vi "Read Measurements.vi"(8 "error in":errorcluster, 9 "Data Frame Format In":T1, 10 "Unit ID (A)":string="A", 11 "VISA Session In":refnum<visa-resource-name>="Alicat") -> (0 "error out":errorcluster, 1 "Data Frame Format Out":T1, 2 "Data Cluster":T2, 3 "VISA Session Out":refnum<visa-resource-name>, 4 "Unknown Dataframe Info":bool, 5 "Error/Overrange/Unknown String":string, 6 "Error Present":bool, 7 "Range Exceeded":bool)   [LabVIEW 2020]
doc: "Polls the Alicat device for its data frame and outputs cluster of data, retrieved/used data flags, and error/overrange/unknown indicators and strings. Data is parsed according to data flag inputs, and if none are present the device will query the data flags (adding a considerable amount of time to the VI's execution)."
uses:
  Data Cluster.ctl
  Data Frame.ctl
  <vilib>/Instr/_visa.llb/VISA Flush IO Buffer Mask.ctl
panel:
  # "Totalizer Timer"
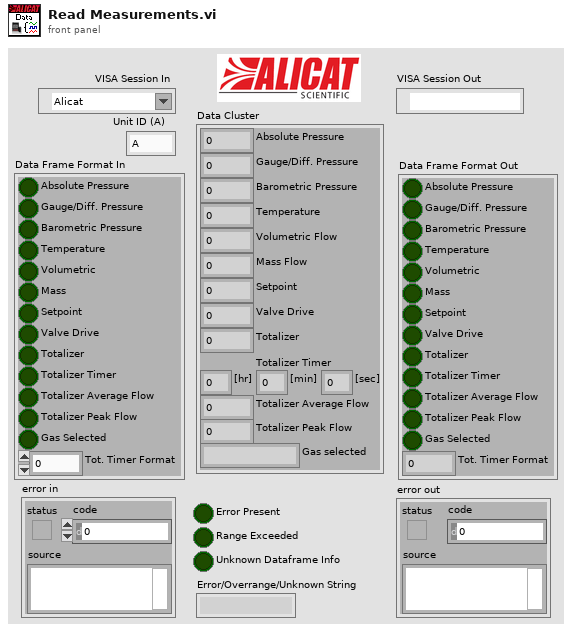
[diagram p1: front panel]
types:
  T1 = typedef "Data Frame.ctl" = cluster{"Absolute Pressure":bool, "Gauge/Diff. Pressure":bool, "Barometric Pressure":bool, "Temperature":bool, "Volumetric":bool, "Mass":bool, "Setpoint":bool, "Valve Drive":bool, "Totalizer":bool, "Totalizer Timer":bool, "Totalizer Average Flow":bool, "Totalizer Peak Flow":bool, "Gas Selected":bool, "Tot. Timer Format":u16}
  T2 = typedef "Data Cluster.ctl" = cluster{"Absolute Pressure":dbl, "Gauge/Diff. Pressure":dbl, "Barometric Pressure":dbl, "Temperature":dbl, "Volumetric Flow":dbl, "Mass Flow":dbl, "Setpoint":dbl, "Valve Drive":dbl, "Totalizer":dbl, "[hr]":dbl, "[min]":dbl, "[sec]":dbl, "Totalizer Average Flow":dbl, "Totalizer Peak Flow":dbl, "Gas selected":string}
  T3 = cluster{"Absolute Pressure":dbl, "Gauge/Diff. Pressure":dbl, "Barometric Pressure":dbl, "Temperature":dbl, "Volumetric":dbl, "Mass":dbl, "Setpoint":dbl, "Valve Drive":dbl, "Totalizer":dbl, "[hr]":dbl, "[min]":dbl, "[sec]":dbl, "Totalizer Average Flow":dbl, "Totalizer Peak Flow":dbl, "Gas selected":string}
  T4 = typedef "VISA Flush IO Buffer Mask.ctl" = u16
  T5 = cluster{"Absolute Pressure":dbl, "Gauge/Diff. Pressure":dbl, "Barometric Pressure":dbl, "Temperature":dbl, "Volumetric Flow":dbl, "Mass Flow":dbl, "Setpoint":dbl, "Valve Drive":dbl, "Totalizer":dbl, "[hr]":dbl, "[min]":dbl, "[sec]":dbl, "Totalizer Average Flow":dbl, "Totalizer Peak Flow":dbl, "Gas selected":string}
  T6 = cluster{"Absolute Pressure":bool, "Gauge/Diff. Pressure":bool, "Barometric Pressure":bool, "Temperature":bool, "Volumetric":bool, "Mass":bool, "Setpoint":bool, "Valve Drive":bool, "Totalizer":bool, "Totalizer Timer":bool, "Totalizer Average Flow":bool, "Totalizer Peak Flow":bool, "Gas Selected":bool, "Tot. Timer Format":u16}
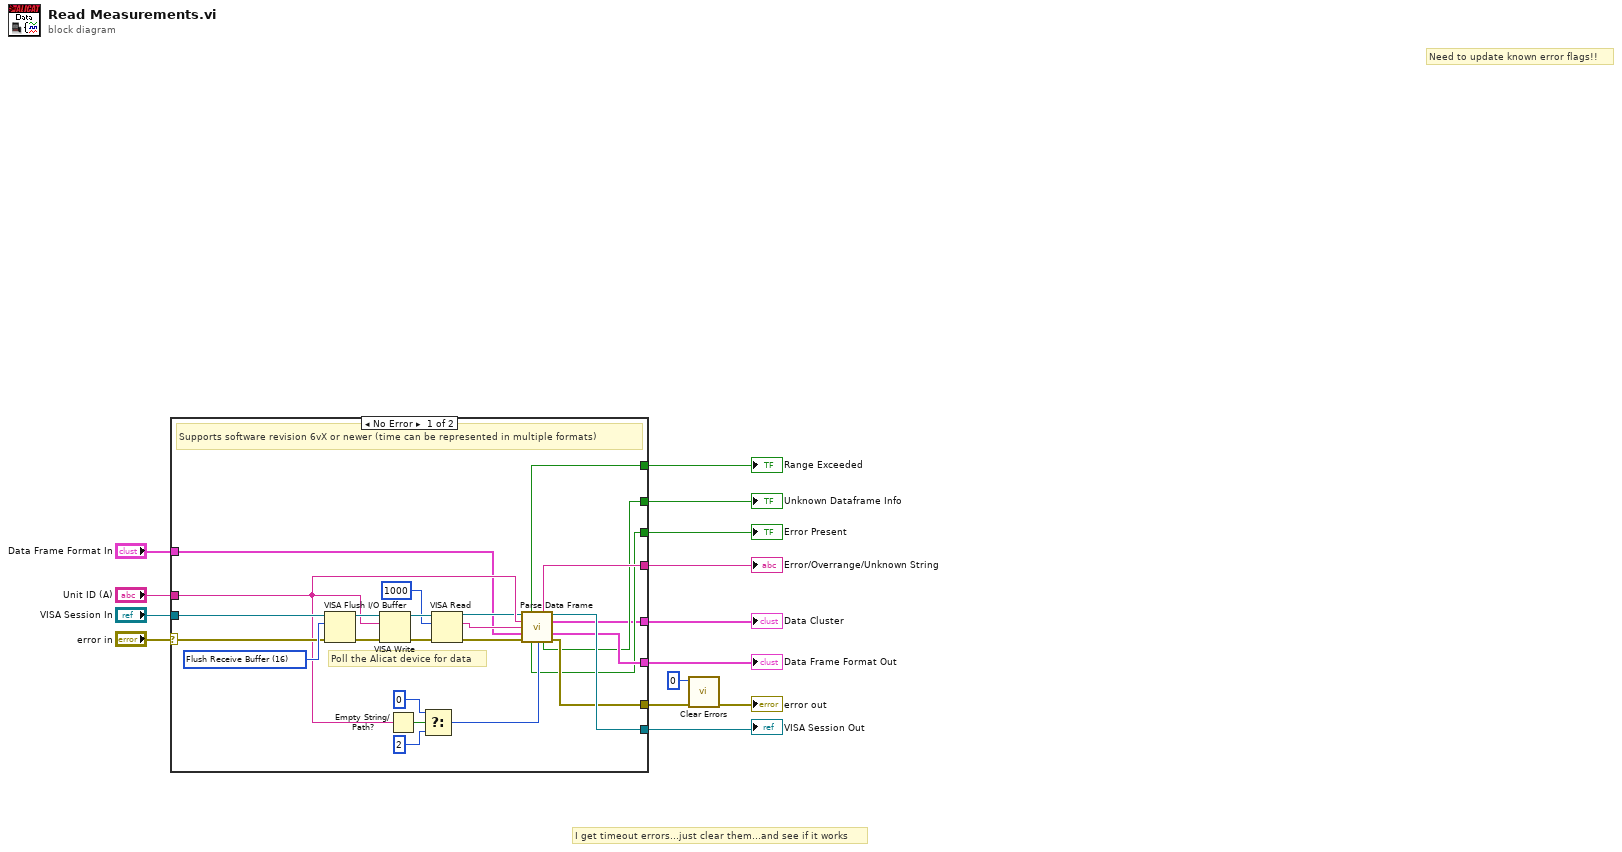
[diagram p0: block diagram]
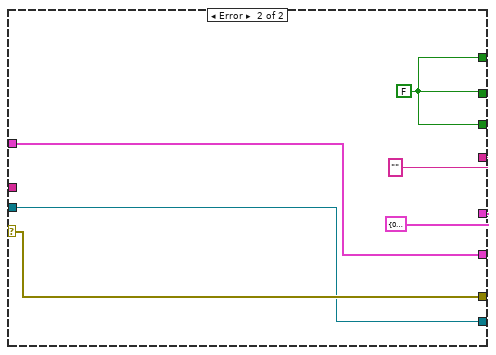
[diagram p2: hidden frame]
diagram:
  # "I get timeout errors...just clear them...and see if it works"
  # "Need to update known error flags!!"
  n1 = case shown="No Error" "error in" {
    selector: "error in" -> [w28 w45]
    tunnel: "VISA Session In" -> [w27 w44]
    tunnel: "Unit ID (A)" -> [w26 _]
    tunnel: [w16 w41] -> w13
    tunnel: [w22 w41] -> w12
    tunnel: [w17 w41] -> w11
    tunnel: [w21 ""] -> w10
    tunnel: [w20 w44] -> w9
    tunnel: [w19 w45] -> w3
    tunnel: "Data Frame Format In" -> [w23 w43]
    tunnel: [w18 w43] -> w5
    tunnel: [w15 T3 {"Absolute Pressure"=0.0, "Gauge/Diff. Pressure"=0.0, "Barometric Pressure"=0.0, "Temperature"=0.0, "Volumetric"=0.0, "Mass"=0.0, "Setpoint"=0.0, "Valve Drive"=0.0, "Totalizer"=0.0, "[hr]"=0.0, "[min]"=0.0, "[sec]"=0.0, "Totalizer Average Flow"=0.0, "Totalizer Peak Flow"=0.0, "Gas selected"=""} ("Data Cluster 2")] -> w8
    frame No Error {
      w34 = T4 16 items=["Flush Receive Buffer"=16, "Write Transmit Buffer to Device"=32, "Flush Receive Buffer (No I/O)"=64, "Flush Transmit Buffer"=128] ("Mask")
      # "Poll the Alicat device for data"
      # "Supports software revision 6vX or newer (time can be represented in multiple formats)"
      n2 = VISA Flush I/O Buffer(VISA resource name=w27, mask (16)=w34, error in (no error)=w28) -> (VISA resource name out=w32:refnum<visa-resource-name>, error out=w30:errorcluster)
      n3 = VISA Write(VISA resource name=w32, write buffer=w26, error in (no error)=w30) -> (VISA resource name out=w33:refnum<visa-resource-name>, error out=w31:errorcluster)  [unwired: 1 out]
      n4 = Empty String/Path?(string/path=w26) -> (empty?=w35:bool)
      n5 = Select(t=u32 0, s=w35, f=u32 2) -> (s? t:f=w38:u32)
      n6 = VISA Read(VISA resource name=w33, byte count=u32 1000, error in (no error)=w31) -> (VISA resource name out=w24:refnum<visa-resource-name>, read buffer=w39:string, error out=w25:errorcluster)  [unwired: 1 out]
      n7 = call "Parse Data Frame.vi"("VISA Session In"=w24, "Unit ID (A)"=w26, "Data Frame Input"=w39, "Data Frame Format In"=w23, "error in"=w25, "Offset (2 if polling, 0 if streaming)"=w38) -> ("Range Exceeded"=w22:bool, "Error/Overrange/Unknown String"=w21:string, "VISA Session Out"=w20:refnum<visa-resource-name>, "Data Cluster"=w15:T5, "Data Frame Format Out"=w18:T6, "Error Present"=w16:bool, "Unknown Dataframe Info"=w17:bool, "error out"=w19:errorcluster)  [unwired: 2 in]
    }
    frame Error {
      w41 = FALSE
    }
  }
  "VISA Session Out" <- w9
  "Error Present" <- w13
  "Range Exceeded" <- w12
  "Unknown Dataframe Info" <- w11
  "Error/Overrange/Unknown String" <- w10
  "Data Cluster" <- w8
  "Data Frame Format Out" <- w5
  n8 = call <vilib>:"Clear Errors.vi"("error in (no error)"=w3, "specific error code to clear (0: all)"=0) -> ("error out"=→"error out":errorcluster)  [unwired: 4 in, 1 out]
